vi "Get Test Number.vi"(8 "error in":errorcluster, 11 "conn":u32) -> (0 "error out":errorcluster, 2 "test_num":i32, 3 "PQresultStatus":T1(ring))   [LabVIEW 2018]
uses:
  PostgreSQL2LabVIEW/libpqlv/libpqlv.lvlib
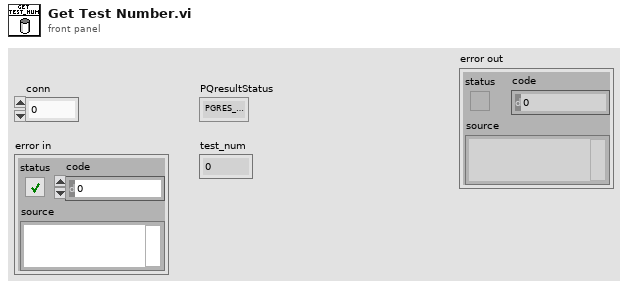
[diagram p1: front panel]
types:
  T1 = enum16{"PGRES_EMPTY_QUERY", "PGRES_COMMAND_OK", "PGRES_TUPLES_OK", "PGRES_COPY_OUT", "PGRES_COPY_IN", "PGRES_BAD_RESPONSE", "PGRES_NONFATAL_ERROR", "PGRES_FATAL_ERROR"}
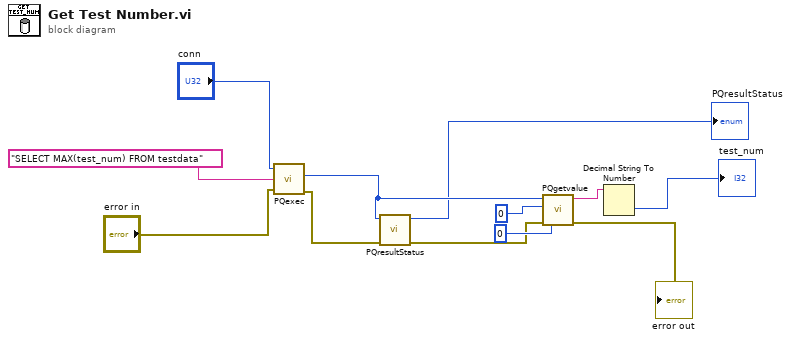
[diagram p0: block diagram]
diagram:
  n1 = call "PQexec.vi"("conn"="conn", "query"="SELECT MAX(test_num) FROM testdata", "error in (no error)"="error in") -> ("PGresult"=w9:u32, "error out"=w10:errorcluster)  [unwired: 2 in]
  n2 = call "PQresultStatus.vi"("error in (no error)"=w10, "res"=w9) -> ("error out"=w6:errorcluster, "PQresultStatus"=→"PQresultStatus":T1)  [unwired: 8 in]
  n3 = call "PQgetvalue.vi"("error in (no error)"=w6, "column_number"=0, "row_number"=0, "res"=w9) -> ("error out"=→"error out":errorcluster, "field_value"=w11:string)  [unwired: 6 in]
  n4 = Decimal String To Number(string=w11) -> (number=→"test_num":i32)  [unwired: 2 in, 1 out]
